vi "Previous Page.vi"(8 "error in (no error)":errorcluster, 11 "Sensor Model in":refnum<class "Sensor Model.lvclass">) -> (0 "error out":errorcluster, 3 "Sensor Model out":refnum<class "Sensor Model.lvclass">)   [LabVIEW 2013, in "Sensor Model.lvlib" / "Sensor Model.lvclass"]
uses:
  Sensor Model.lvclass
  Sensor Model.lvclass/Sensor Model.ctl
  <vilib>/ActorFrameworkMVC/View Observer/View Registry/View Registry.lvclass/View Registry.ctl
  Sensor Model Messages/Abstract Sensor Move In Previous Msg/Abstract Sensor Move In Previous Msg.lvclass
  <vilib>/ActorFrameworkMVC/View Observer/Data Message/Data Message.lvclass
  <vilib>/ActorFrameworkMVC/View Observer/View Registry/View Registry.lvclass
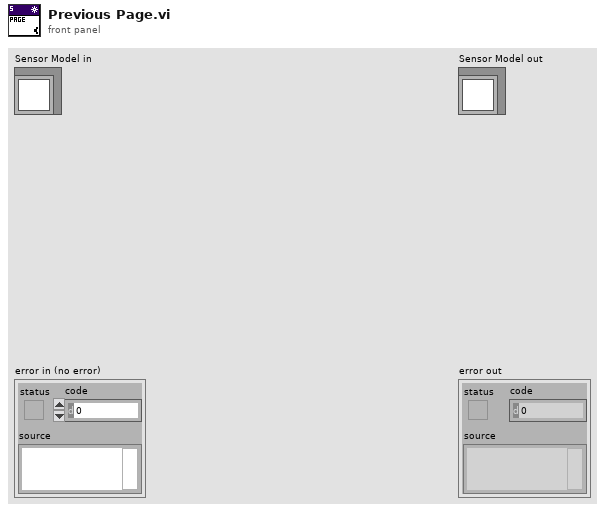
[diagram p1: front panel]
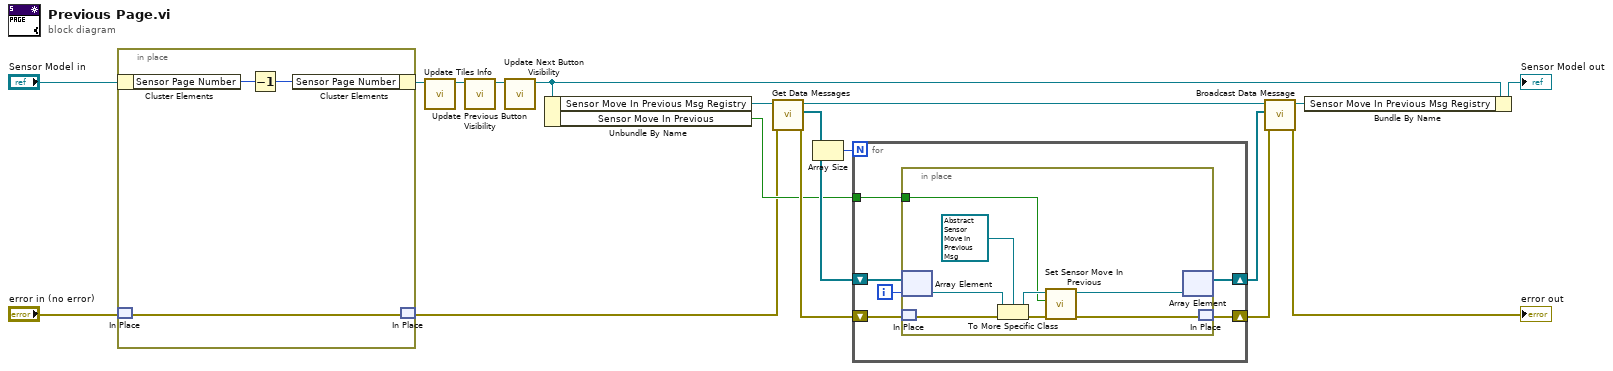
[diagram p0: block diagram]
diagram:
  n1 = in-place {
    n2 = in-place-cluster #1("Sensor Model in") -> ("Sensor Page Number"=w21:i32)
    n3 = in-place-match #2("error in (no error)") -> (w19:errorcluster)
    n4 = Decrement(x=w21) -> (x-1=w20:i32)
    n5 = in-place-cluster #1("Sensor Page Number"=w20) -> (w7:refnum<class "Sensor Model.lvclass">)
    n6 = in-place-match #2(w19) -> (w4:errorcluster)
  }
  n7 = call "Update Tiles Info.vi"("Sensor Model in"=w7) -> ("Sensor Model out"=w3:refnum<class "Sensor Model.lvclass">)  [unwired: 9 in, 1 out]
  n8 = call "Update Previous Button Visibility.vi"("Sensor Model in"=w3) -> ("Sensor Model out"=w2:refnum<class "Sensor Model.lvclass">)  [unwired: 9 in, 1 out]
  n9 = call "Update Next Button Visibility.vi"("Sensor Model in"=w2) -> ("Sensor Model out"=w1:refnum<class "Sensor Model.lvclass">)  [unwired: 9 in, 1 out]
  n10 = Unbundle By Name(w1) -> ("Sensor Move In Previous Msg Registry"=w16:refnum<class "View Registry.lvclass">, "Sensor Move In Previous"=w8:bool)
  n11 = call <vilib>:"Get Data Messages.vi"("error in (no error)"=w4, "View Registry in"=w16) -> ("error out"=w12:errorcluster, "Data Messages"=w13:refnum<class "Data Message.lvclass">[], "View Registry out"=w15:refnum<class "View Registry.lvclass">)  [unwired: 7 in]
  n12 = Array Size(array=w13) -> (size(s)=w14:i32)
  n13 = for {
    N: w14 -> [_]
    shift-right: [w26] -> w11
    shift-left: w13 -> [w27]
    shift-right: [w23] -> w10
    shift-left: w12 -> [w25]
    tunnel: w8 -> [w24]
    i -> [w22]
    n14 = in-place {
      in-place-border: w24 -> [w28]
      n15 = in-place-array #3(w27, w22) -> (w33:refnum<class "Data Message.lvclass">)
      n16 = in-place-match #4(w25) -> (w35:errorcluster)
      n17 = To More Specific Class(target class=refnum<class "Abstract Sensor Move In Previous Msg.lvclass"> refnum ("Sensor Model.lvlib:Abstract Sensor Move In Previous Msg.lvclass"), reference=w33, error in=w35) -> (specific class reference=w29:refnum<class "Abstract Sensor Move In Previous Msg.lvclass">, error out=w32:errorcluster)
      n18 = call "Set Sensor Move In Previous.vi"("error in (no error)"=w32, "Sensor Move In Previous"=w28, "Abstract Sensor Move In Previous Msg in"=w29) -> ("error out"=w31:errorcluster, "Abstract Sensor Move In Previous Msg out"=w30:refnum<class "Abstract Sensor Move In Previous Msg.lvclass">)  [unwired: 7 in]
      n19 = in-place-array #3(w30) -> (w26:refnum<class "Data Message.lvclass">[])  [unwired: 1 out]
      n20 = in-place-match #4(w31) -> (w23:errorcluster)
    }
  }
  n21 = call <vilib>:"Broadcast Data Message.vi"("error in (no error)"=w10, "Data Messages"=w11, "View Registry in"=w15) -> ("error out"=→"error out":errorcluster, "View Registry out"=w9:refnum<class "View Registry.lvclass">)  [unwired: 7 in]
  n22 = Bundle By Name(cluster=w1, "Sensor Move In Previous Msg Registry"=w9) -> (→"Sensor Model out":refnum<class "Sensor Model.lvclass">)
